vi "禹山探头校准.vi"(5 "校准方式":u16, 6 "MB_Master输入":refnum<class "MB_Master.lvclass">, 7 "探头":T1(ring), 8 "错误输入（无错误）":errorcluster, 9 "标液三":cluster{"标准值":dbl, "检测值":dbl, "原始值":dbl}, 10 "标液二":cluster{"标准值":dbl, "检测值":dbl, "原始值":dbl}, 11 "标液一":cluster{"标准值":dbl, "检测值":dbl, "原始值":dbl}) -> (0 "错误输出":errorcluster)   [LabVIEW 2016, in "斯坦道多参数.lvlib"]
uses:
  <vilib>/Plasmionique/MB Master/MB_Master/MB_Master.lvclass
  <vilib>/Analysis/NI_AALPro.lvlib
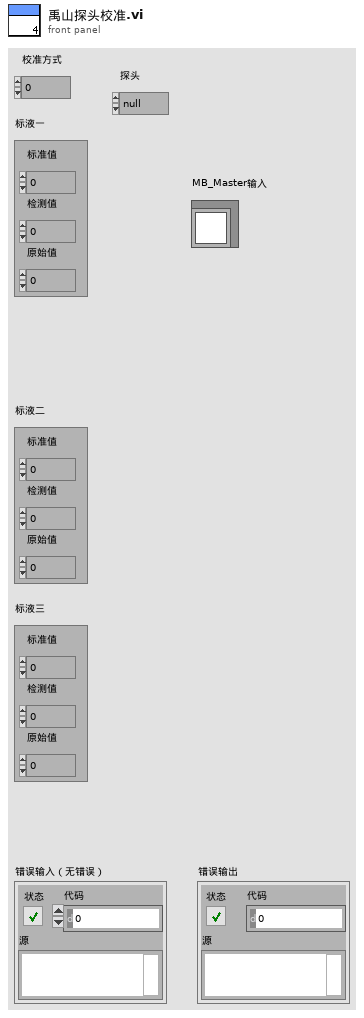
[diagram p1: front panel]
types:
  T1 = enum16{"null", "pH", "DO", "浊度", "电导率", "叶绿素a", "DO2"}
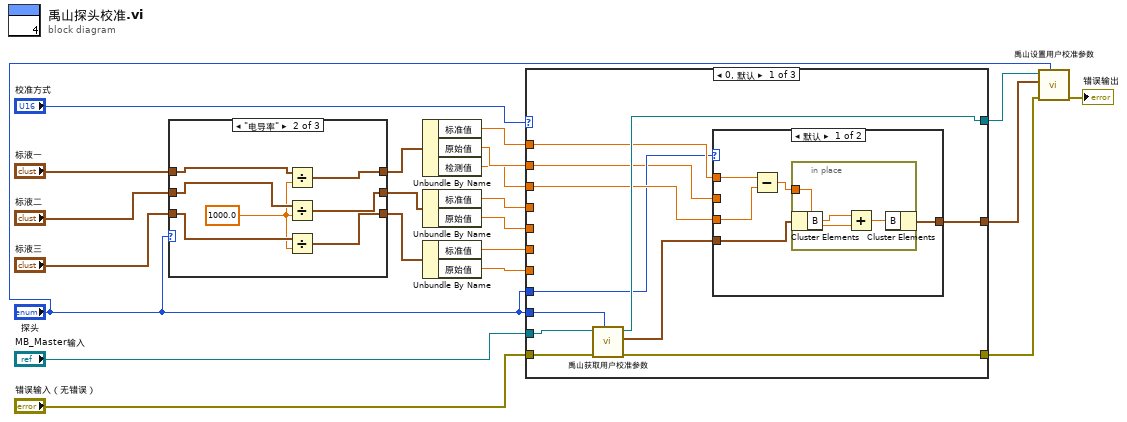
[diagram p0: block diagram]
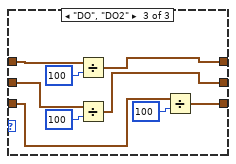
[diagram p3: hidden frame]
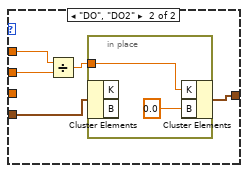
[diagram p4: hidden frame]
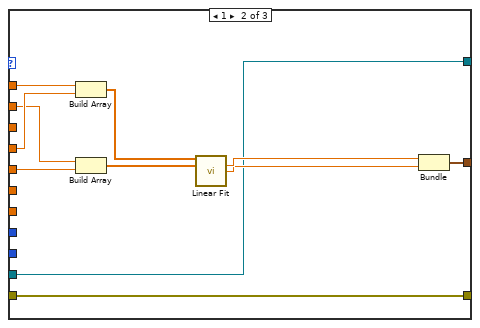
[diagram p5: hidden frame]
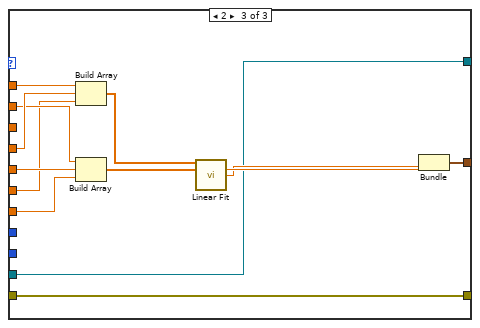
[diagram p6: hidden frame]
diagram:
  n1 = case shown="\"电导率\"" "探头" {
    tunnel: "标液三" -> [w22 w27 w40]
    tunnel: "标液二" -> [w23 w29 w39]
    tunnel: "标液一" -> [w24 w31 w38]
    tunnel: [w24 w30 w37] -> w5
    tunnel: [w23 w28 w35] -> w4
    tunnel: [w22 w26 w33] -> w3
    frame "null", Default {
    }
    frame "电导率" {
      w25 = 1000.0
      n2 = Divide(x=w31, y=w25) -> (x/y=w30:cluster{"标准值":dbl, "检测值":dbl, "原始值":dbl})
      n3 = Divide(x=w29, y=w25) -> (x/y=w28:cluster{"标准值":dbl, "检测值":dbl, "原始值":dbl})
      n4 = Divide(x=w27, y=w25) -> (x/y=w26:cluster{"标准值":dbl, "检测值":dbl, "原始值":dbl})
    }
    frame "DO", "DO2" {
      n5 = Divide(x=w38, y=100) -> (x/y=w37:cluster{"标准值":dbl, "检测值":dbl, "原始值":dbl})
      n6 = Divide(x=w39, y=100) -> (x/y=w35:cluster{"标准值":dbl, "检测值":dbl, "原始值":dbl})
      n7 = Divide(x=w40, y=100) -> (x/y=w33:cluster{"标准值":dbl, "检测值":dbl, "原始值":dbl})
    }
  }
  n8 = Unbundle By Name(w5) -> ("标准值"=w15:dbl, "原始值"=w16:dbl, "检测值"=w2:dbl)
  n9 = Unbundle By Name(w4) -> ("标准值"=w18:dbl, "原始值"=w19:dbl)
  n10 = Unbundle By Name(w3) -> ("标准值"=w20:dbl, "原始值"=w21:dbl)
  n11 = case shown="0, 默认" "校准方式" {
    tunnel: "MB_Master输入" -> [w51 w68 w81]
    tunnel: [w50 w68 w81] -> w7
    tunnel: [w49 w67 w80] -> w9
    tunnel: [w47 w69 w82] -> w11
    tunnel: "错误输入（无错误）" -> [w46 w67 w80]
    tunnel: w15 -> [w45 w77 w90]
    tunnel: w16 -> [w41 w75 w88]
    tunnel: w18 -> [_ w76 w89]
    tunnel: w19 -> [_ w74 w87]
    tunnel: w20 -> [_ _ w79]
    tunnel: w21 -> [_ _ w78]
    tunnel: "探头" -> [w44 _ _]
    tunnel: w2 -> [w43 _ _]
    tunnel: "探头" -> [w42 _ _]
    frame 0, Default {
      n12 = call "禹山获取用户校准参数.vi"("探头"=w44, "error in (no error)"=w46, "MB session in"=w51) -> ("error out"=w49:errorcluster, "输出值"=w48:cluster{"K":sgl, "B":sgl}, "MB session out"=w50:refnum<class "MB_Master.lvclass">)  [unwired: 6 in]
      n13 = case shown="默认" w42 {
        tunnel: w48 -> [w56 w64]
        tunnel: [w55 w63] -> w47
        tunnel: w45 -> [w54 w61]
        tunnel: w43 -> [w52 _]
        tunnel: w41 -> [_ w60]
        frame Default {
          n14 = Subtract(x=w54, y=w52) -> (x-y=w53:dbl)
          n15 = in-place {
            in-place-border: w53 -> [w59]
            n16 = in-place-cluster #1(w56) -> ("B"=w57:sgl)
            n17 = Add(x=w57, y=w59) -> (x+y=w58:dbl)
            n18 = in-place-cluster #1("B"=w58) -> (w55:cluster{"K":sgl, "B":sgl})
          }
        }
        frame "DO", "DO2" {
          n19 = Divide(x=w61, y=w60) -> (x/y=w62:dbl)
          n20 = in-place {
            in-place-border: w62 -> [w66]
            n21 = in-place-cluster #2(w64) -> ()  [unwired: 2 out]
            n22 = in-place-cluster #2("K"=w66, "B"=sgl 0.0) -> (w63:cluster{"K":sgl, "B":sgl})
          }
        }
      }
    }
    frame 1 {
      n23 = Build Array(w77, w76) -> (w73:dbl[])
      n24 = Build Array(w75, w74) -> (w72:dbl[])
      n25 = call <vilib>:"Linear Fit.vi"("Y"=w73, "X"=w72) -> ("slope"=w71:dbl, "intercept"=w70:dbl)  [unwired: 9 in, 3 out]
      n26 = Bundle("slope"=w71, "intercept"=w70) -> (w69:cluster{"slope":dbl, "intercept":dbl})  [unwired: 1 in]
    }
    frame 2 {
      n27 = Build Array(w90, w89, w79) -> (w86:dbl[])
      n28 = Build Array(w88, w87, w78) -> (w85:dbl[])
      n29 = call <vilib>:"Linear Fit.vi"("Y"=w86, "X"=w85) -> ("slope"=w84:dbl, "intercept"=w83:dbl)  [unwired: 9 in, 3 out]
      n30 = Bundle("slope"=w84, "intercept"=w83) -> (w82:cluster{"slope":dbl, "intercept":dbl})  [unwired: 1 in]
    }
  }
  n31 = call "禹山设置用户校准参数.vi"("探头"="探头", "error in (no error)"=w9, "用户校准参数"=w11, "MB session in"=w7) -> ("error out"=→"错误输出":errorcluster)  [unwired: 6 in, 1 out]
